vi "Feature Vector State Action.vi"(10 "action":dbl, 11 "state":dbl[](array[numeric])=[0.46211715726000974, 0.46211715726000974, 0.7071067811865475]) -> (3 "x(s, a)":dbl[](array[numeric])=[1.0, -0.6056998670788134, -0.26625534204141565, 0.11873171128012475, -0.8619805458075959, 0.9254712927602428, -0.9718055614729862, 0.40101101649098936])   [LabVIEW 2017]
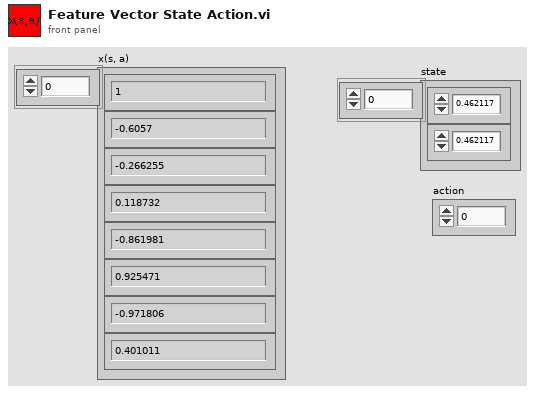
[diagram p1: front panel]
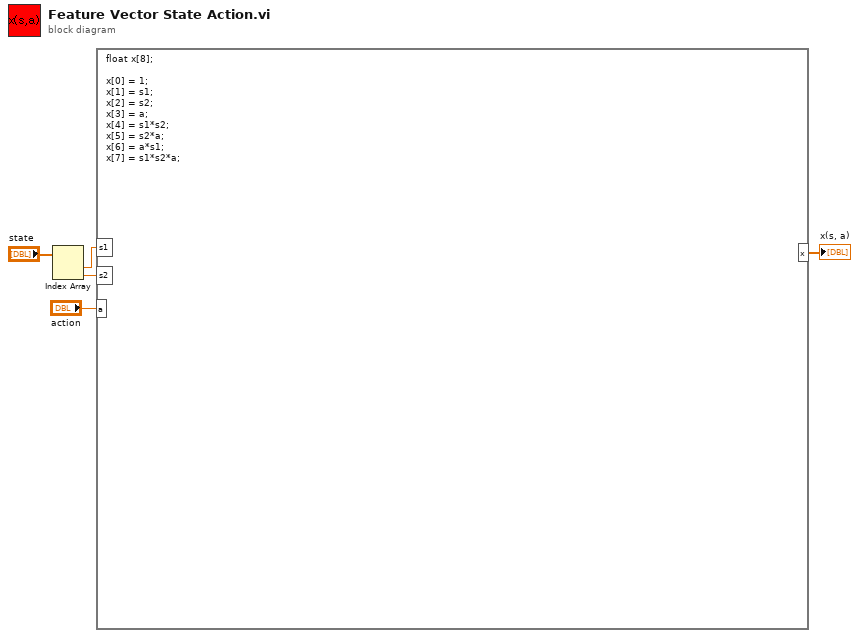
[diagram p0: block diagram]
diagram:
  n1 = Index Array(array="state") -> (element #1=w4:dbl, element #2=w3:dbl)  [unwired: 2 in]
  n2 = formula code="float x[8];\n\nx[0] = 1;\nx[1] = s1;\nx[2] = s2;\nx[3] = a;\nx[4] = s1*s2;\nx[5] = s2*a;\nx[6] = a*s1;\nx[7] = s1*s2*a;"("s1"=w4, "s2"=w3, "a"="action") -> ("x"=→"x(s, a)":dbl[])
